vi "Capacitance_ProcessingData.vi"(6 "Measure Record dt":dbl, 8 "current measurements":dbl[](array[numeric]), 9 "voltage measurements":dbl[](array[numeric]), 10 "RecordLength":i32, 11 "DCPower_SequenceParameters":T1 {"DeltaVoltage" format="%.6p"; "DeltaTime" format="%.6p"; "Voltage Stop" format="%.6p"; "Aperture_time" format="%.6p"; "Current_range" format="%.6p"; "Current" format="%.6p"; "Voltage_range" format="%.6p"; "Voltage Start" format="%.6p"}) -> (3 "Capacitance":dbl)   [LabVIEW 2023, in "Capacitance.lvlib"]
uses:
  Capacitance.lvlib
  ResourceHandling/TypeDefs/RH_DCPower_SequenceParameters.ctl
  <vilib>/Analysis/baseanly.llb/Mean (DBL).vi
  <vilib>/Analysis/NI_AALBase.lvlib
  ResourceHandling/ResourceHandling.lvlib
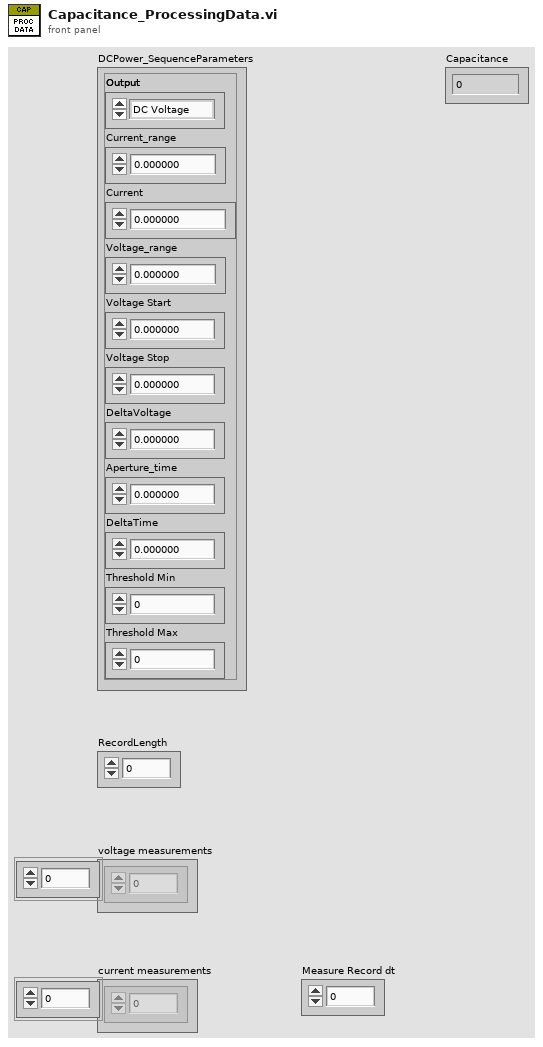
[diagram p1: front panel]
types:
  T1 = typedef "ResourceHandling.lvlib/RH_DCPower_SequenceParameters.ctl" = cluster{"Output":enum16{"DC Voltage", "DC Current"}, "Current_range":dbl, "Current":dbl, "Voltage_range":dbl, "Voltage Start":dbl, "Voltage Stop":dbl, "DeltaVoltage":dbl, "Aperture_time":dbl, "DeltaTime":dbl, "Threshold Min":dbl, "Threshold Max":dbl}
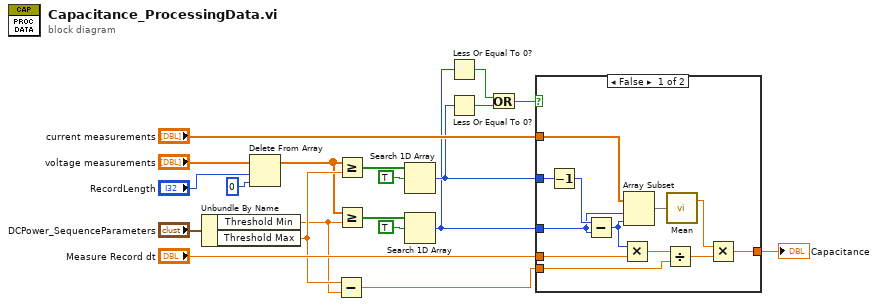
[diagram p0: block diagram]
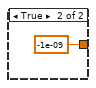
[diagram p2: hidden frame]
diagram:
  n1 = Unbundle By Name("DCPower_SequenceParameters") -> ("Threshold Min"=w14:dbl, "Threshold Max"=w15:dbl)
  n2 = Delete From Array(array="voltage measurements", length="RecordLength", index=0) -> (array with subset deleted=w13:dbl[])  [unwired: 1 out]
  n3 = Subtract(x=w15, y=w14) -> (x-y=w6:dbl)
  n4 = Greater Or Equal?(x=w13, y=w15) -> (x >= y?=w17:bool[])
  n5 = Greater Or Equal?(x=w13, y=w14) -> (x >= y?=w16:bool[])
  n6 = Search 1D Array(1D array=w17, element=TRUE) -> (index of element=w8:i32)  [unwired: 1 in]
  n7 = Search 1D Array(1D array=w16, element=TRUE) -> (index of element=w7:i32)  [unwired: 1 in]
  n8 = Less Or Equal To 0?(x=w7) -> (x <= 0?=w9:bool)
  n9 = Less Or Equal To 0?(x=w8) -> (x <= 0?=w10:bool)
  n10 = Or(x=w9, y=w10) -> (x .or. y?=w11:bool)
  n11 = case shown="False" w11 {
    tunnel: w8 -> [w32 _]
    tunnel: w6 -> [w29 _]
    tunnel: w7 -> [w27 _]
    tunnel: [w24 -1e-09] -> w20
    tunnel: "current measurements" -> [w23 _]
    tunnel: "Measure Record dt" -> [w21 _]
    frame False {
      n12 = Decrement(x=w32) -> (x-1=w31:i32)
      n13 = Subtract(x=w31, y=w27) -> (x-y=w26:i32)
      n14 = Multiply(x=w26, y=w21) -> (x*y=w30:dbl)
      n15 = Array Subset(array=w23, index=w27, length=w26) -> (w22:dbl[])
      n16 = Divide(x=w30, y=w29) -> (x/y=w28:dbl)
      n17 = call-poly <vilib>:"Mean.vi"("X"=w22) -> ("mean"=w25:dbl)  [unwired: 1 out]
      n18 = Multiply(x=w25, y=w28) -> (x*y=w24:dbl)
    }
    frame True {
    }
  }
  "Capacitance" <- w20
